vi "Launch VI in Project Instance.vi"(8 "error in (no error)":errorcluster, 10 "VI Path":path, 11 "Project Path":path) -> (0 "error out":errorcluster)   [LabVIEW 2014, in "SLL Application.lvlib"]
doc: "Launches a VI in a project instance whose project path is specified"
uses:
  SLL Application.lvlib
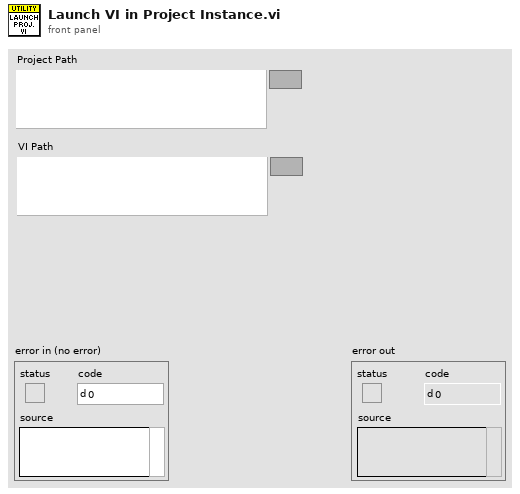
[diagram p1: front panel]
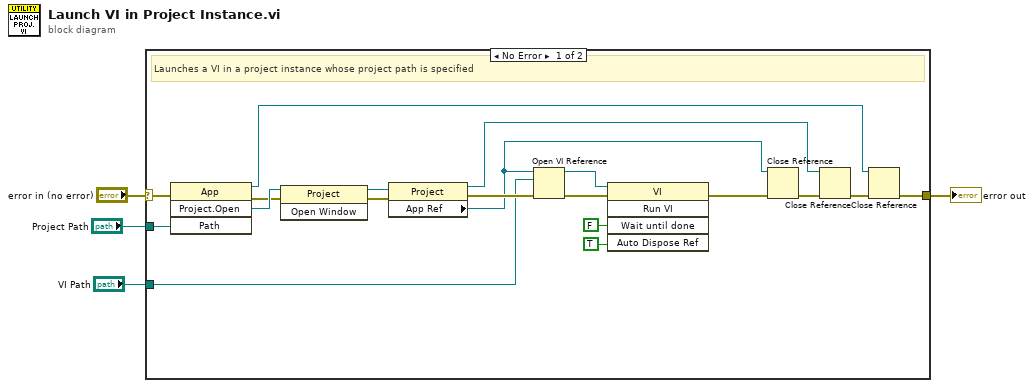
[diagram p0: block diagram]
diagram:
  n1 = case shown="No Error" "error in (no error)" {
    selector: "error in (no error)" -> [w23 w24]
    tunnel: [w6 w24] -> w3
    tunnel: "Project Path" -> [w22 _]
    tunnel: "VI Path" -> [w20 _]
    frame No Error {
      # "Launches a VI in a project instance whose project path is specified"
      n2 = invoke class="App" method="Project.Open"(error in=w23, "Path"=w22) -> (reference out=w5:refnum<vi>, error out=w9:errorcluster, "Project:Open"=w11:refnum<vi>)  [unwired: 2 in, 1 out]
      n3 = invoke class="Project" method="Open Window"(reference=w11, error in=w9) -> (reference out=w10:refnum<vi>, error out=w8:errorcluster)  [unwired: 1 in, 1 out]
      n4 = property class="Project"(reference=w10, error in=w8) -> (reference out=w12:refnum<vi>, error out=w21:errorcluster, "App Ref"=w14:refnum<vi>)
      n5 = Open VI Reference(application reference (local)=w14, vi path=w20, error in (no error)=w21) -> (vi reference=w17:refnum<vi>, error out=w19:errorcluster)  [unwired: 3 in]
      n6 = invoke class="VI" method="Run VI"(reference=w17, error in=w19, "Wait until done"=FALSE ("Wait Until Done"), "Auto Dispose Ref"=TRUE ("Auto Dispose Reference")) -> (error out=w18:errorcluster)  [unwired: 1 in, 4 out]
      n7 = Close Reference(reference=w14, error in (no error)=w18) -> (error out=w13:errorcluster)
      n8 = Close Reference(reference=w12, error in (no error)=w13) -> (error out=w7:errorcluster)
      n9 = Close Reference(reference=w5, error in (no error)=w7) -> (error out=w6:errorcluster)
    }
    frame Error {
    }
  }
  "error out" <- w3
